vi "Lab Panel V5.28.vi"() -> ()   [LabVIEW 2013] (continued)
                  tunnel: w845 -> [_ w883]
                  tunnel: w844 -> [_ w882]
                  tunnel: w842 -> [w847 w881]
                  tunnel: w843 -> [_ w880]
                  tunnel: w841 -> [_ w879]
                  tunnel: [w846 w878] -> w840
                  tunnel: w838 -> [_ w877]
                  tunnel: w837 -> [_ w876]
                  tunnel: w836 -> [_ w875]
                  tunnel: w835 -> [_ w873]
                  frame False {
                    # "stop test"
                    n579 = stacked-sequence {
                      tunnel: w847 -> [w856 _]
                      tunnel: [w848 _] -> w846
                      frame #0 {
                        n580 = local read "DISP LAB01-2"() -> (w855:T4)
                        n581 = Unbundle(w855) -> ("CYCLE"=w853:dbl, "MINS"=w854:dbl)  [unwired: 1 out]
                        n582 = case shown="\"CHART TEST\", Default" w856 {
                          tunnel: w854 -> [_ _ w863]
                          tunnel: w853 -> [w861 w862 _]
                          tunnel: [w861 w862 w863] -> w852
                          frame "CHART TEST", Default {
                          }
                          frame "CYCLE TEST" {
                          }
                          frame "T-RISE TEST" {
                          }
                        }
                        n583 = local read "TDMS LAB01-2"() -> (w860:refnum<k34>)
                        n584 = Build Array("STOPPED") -> (w857:string[])
                        n585 = Build Array(w852) -> (w851:dbl[])
                        n586 = TDMS Write(0:w860, 5:"TEST RESULT", 7:w857, 9:w851) -> (4:w849:refnum<k34>, 15:w850:errorcluster)  [unwired: 2 in, 2 out]
                        n587 = TDMS Close(8:w850, 11:w849) -> (0:w848:errorcluster)  [unwired: 1 out]
                      }
                      frame #1 {
                        n588 = local read "DISP LAB01-2"() -> (w867:T4)
                        n589 = stacked-sequence {
                          tunnel: "LAB01-2" -> [w869 w871]
                          frame #0 {
                            n590 = call "sub vi - defrag tdms v1.vi"("panel id"=w869) -> ("error out"=w868:errorcluster)  [unwired: 10 in]
                            n591 = local write "data file error"(w868) -> ()
                          }
                          frame #1 {
                            n592 = call "Save data file (stop) v3.vi"("panel id"=w871) -> ("network file save error"=w870:errorcluster)  [unwired: 9 in, 1 out]
                            n593 = local write "RESULT LAB01-2"(FALSE) -> ()
                            n594 = local write "data file error"(w870) -> ()
                          }
                        }
                        n595 = Bundle(cluster=w867, "STATUS"="STOP") -> (w865:T4)  [unwired: 2 in]
                        n596 = local write "DISP LAB01-2"(w865) -> ()
                      }
                    }
                  }
                  frame True {
                    n597 = local read "SIG LAB01-2"() -> (w874:T2)
                    n598 = stacked-sequence {
                      seq-local: [w885 _] -> [_ w889]
                      tunnel: w883 -> [_ w899]
                      tunnel: w882 -> [_ w898]
                      tunnel: w881 -> [_ w897]
                      tunnel: w880 -> [_ w896]
                      tunnel: w879 -> [_ w895]
                      tunnel: [_ w894] -> w878
                      tunnel: w877 -> [_ w893]
                      tunnel: w876 -> [_ w892]
                      tunnel: w875 -> [_ w891]
                      tunnel: w874 -> [w884 w890]
                      tunnel: w873 -> [_ w888]
                      frame #0 {
                        n599 = Unbundle(w884) -> ("AMPS"=w887:dbl)  [unwired: 4 out]
                        n600 = call "Check For Amps on v1.vi"("ID"="LAB01-2", "amps"=w887) -> ("amps"=w885:bool)  [unwired: 9 in]
                      }
                      frame #1 {
                        n601 = case shown="True" w889 {
                          tunnel: w899 -> [_ w912]
                          tunnel: w898 -> [_ w911]
                          tunnel: w897 -> [_ w910]
                          tunnel: w896 -> [_ w909]
                          tunnel: w895 -> [_ w908]
                          tunnel: [errorcluster {"status"=FALSE, "code"=0, "source"=""} ("error out") w907] -> w894
                          tunnel: w893 -> [_ w906]
                          tunnel: w892 -> [_ w905]
                          tunnel: w891 -> [_ w904]
                          tunnel: w890 -> [_ w903]
                          tunnel: w888 -> [_ w902]
                          frame False {
                            w900 = FALSE
                            n602 = local write "RUN LAB01-2"(w900) -> ()
                            n603 = local write "run lab01-2"(w900) -> ()
                          }
                          frame True {
                            n604 = stacked-sequence {
                              seq-local: [w913 _ _ _ _] -> [_ w937 _ _ _]
                              tunnel: w912 -> [w918 _ _ _ _]
                              tunnel: w911 -> [w915 _ _ _ _]
                              tunnel: w910 -> [w928 _ _ _ _]
                              tunnel: w909 -> [w921 _ _ _ _]
                              tunnel: w908 -> [w916 _ _ _ _]
                              tunnel: [_ w932 _ _ _] -> w907
                              tunnel: w906 -> [_ _ _ w959 _]
                              tunnel: w905 -> [_ _ _ w958 _]
                              tunnel: w904 -> [_ _ _ w957 _]
                              tunnel: w903 -> [_ _ _ _ _]
                              tunnel: w902 -> [_ _ _ _ w972]
                              frame #0 {
                                w914 = "\\"
                                n605 = local read "SET LAB01-2"() -> (w923:T5)
                                n606 = case shown="\"CYCLE TEST\"" w928 {
                                tunnel: ["L01-2-CHART TEST-" "L01-2-CYCLE TEST-" "L01-2-T-RISE TEST-"] -> w924
                                frame "CHART TEST", Default {
                                }
                                frame "CYCLE TEST" {
                                }
                                frame "T-RISE TEST" {
                                }
                                }
                                n607 = Unbundle(w923) -> ("DESCRIPTION"=w922:string)  [unwired: 4 out]
                                n608 = Concatenate Strings(w918, "\\", w916, w914, w915, w914) -> (w925:string)
                                n609 = String To Path(string=w925) -> (path=w927:path)
                                n610 = Concatenate Strings(w925, w924, w922, "-", w921, ".tdms") -> (w913:string)
                                n611 = Create Folder(path (use dialog)=w927) -> (error out=w926:errorcluster)  [unwired: 2 in, 2 out]
                                n612 = call <vilib>:"Clear Errors.vi"("error in (no error)"=w926) -> ()  [unwired: 6 in, 1 out]
                                n613 = global write "Global 1.vi" "LAB01-2 FILE"(w913) -> ()
                              }
                              frame #1 {
                                (unwired) FALSE
                                n614 = String To Path(string=w937) -> (path=w933:path)
                                n615 = TDMS Open(6:FALSE, 10:T21."create or replace" ("operation (0:open)"), 11:w933) -> (0:w932:errorcluster, 3:→"TDMS LAB01-2":refnum<k34>)  [unwired: 4 in]
                              }
                              frame #2 {
                                n616 = local read "SET LAB01-2"() -> (w943:T5)
                                n617 = local read "TDMS LAB01-2"() -> (w954:refnum<k34>)
                                n618 = Build Array("Testers Name", "Description", "Set Test Cycles", "T-Rise minutes", "T-Rise Deg C") -> (w944:string[])
                                n619 = Unbundle(w943) -> ("NAME"=w942:string, "DESCRIPTION"=w941:string, "CYCLES"=w940:dbl, "T-RISE mins"=w939:dbl, "T-RISE deg C"=w938:dbl)
                                n620 = Number To Decimal String(number=w940) -> (decimal integer string=w953:string)  [unwired: 1 in]
                                n621 = Number To Decimal String(number=w939) -> (decimal integer string=w952:string)  [unwired: 1 in]
                                n622 = Number To Decimal String(number=w938) -> (decimal integer string=w951:string)  [unwired: 1 in]
                                n623 = Build Array(w942, w941, w953, w952, w951) -> (w950:string[])
                                n624 = TDMS Set Properties(5:w950, 7:w944, 11:w954) -> ()  [unwired: 3 in, 4 out]
                              }
                              frame #3 {
                                n625 = local read "DISP LAB01-2"() -> (w956:T4)
                                n626 = Concatenate Strings("LAB01-2  ", w959) -> (w960:string)
                                n627 = Two Button Dialog(message=w960, 1:w957, 2:w958) -> (T button?=w962:bool)
                                n628 = case shown="True" w962 {
                                tunnel: w956 -> [w969 w970]
                                tunnel: [w969 w970] -> w966
                                tunnel: [w968 w971] -> w965
                                tunnel: [w967 w971] -> w964
                                frame False {
                                n629 = Unbundle(w969) -> ("CYCLE"=w968:dbl, "MINS"=w967:dbl)  [unwired: 1 out]
                                }
                                frame True {
                                w971 = 0.0
                                }
                                }
                                n630 = Bundle(cluster=w966, "CYCLE"=w965, "MINS"=w964, "STATUS"="RUN") -> (w955:T4)
                                n631 = local write "DISP LAB01-2"(w955) -> ()
                              }
                              frame #4 {
                                n632 = local read "TEMP START LAB01-2"() -> (w974:cluster{"TL":dbl, "TN":dbl})
                                n633 = Bundle(cluster=w974, "TL"=w972, "TN"=w972) -> (w973:cluster{"TL":dbl, "TN":dbl})
                                n634 = local write "TEMP START LAB01-2"(w973) -> ()
                              }
                            }
                          }
                        }
                      }
                    }
                  }
                }
              }
              event "RUN LAB02-1": Value Change {
                n635 = event-data() -> ("NewVal"=w980:bool)  [unwired: 1 in, 5 out]
                n636 = local read "SIG LAB02-1"() -> (w976:T2)
                n637 = case shown="True" w980 {
                  tunnel: w986 -> [_ w1024]
                  tunnel: w985 -> [_ w1023]
                  tunnel: w983 -> [w988 w1022]
                  tunnel: w984 -> [_ w1021]
                  tunnel: w982 -> [_ w1020]
                  tunnel: [w987 w1019] -> w981
                  tunnel: w979 -> [_ w1018]
                  tunnel: w978 -> [_ w1017]
                  tunnel: w977 -> [_ w1016]
                  tunnel: w976 -> [_ w1015]
                  tunnel: w975 -> [_ w1014]
                  frame False {
                    # "stop test"
                    n638 = stacked-sequence {
                      tunnel: w988 -> [w997 _]
                      tunnel: [w989 _] -> w987
                      frame #0 {
                        n639 = local read "DISP LAB02-1"() -> (w996:T4)
                        n640 = Unbundle(w996) -> ("CYCLE"=w994:dbl, "MINS"=w995:dbl)  [unwired: 1 out]
                        n641 = case shown="\"CYCLE TEST\"" w997 {
                          tunnel: w995 -> [_ _ w1004]
                          tunnel: w994 -> [w1002 w1003 _]
                          tunnel: [w1002 w1003 w1004] -> w993
                          frame "CHART TEST", Default {
                          }
                          frame "CYCLE TEST" {
                          }
                          frame "T-RISE TEST" {
                          }
                        }
                        n642 = local read "TDMS LAB02-1"() -> (w1001:refnum<k34>)
                        n643 = Build Array("STOPPED") -> (w998:string[])
                        n644 = Build Array(w993) -> (w992:dbl[])
                        n645 = TDMS Write(0:w1001, 5:"TEST RESULT", 7:w998, 9:w992) -> (4:w990:refnum<k34>, 15:w991:errorcluster)  [unwired: 2 in, 2 out]
                        n646 = TDMS Close(8:w991, 11:w990) -> (0:w989:errorcluster)  [unwired: 1 out]
                      }
                      frame #1 {
                        n647 = local read "DISP LAB02-1"() -> (w1008:T4)
                        n648 = stacked-sequence {
                          tunnel: "LAB02-1" -> [w1010 w1012]
                          frame #0 {
                            n649 = call "sub vi - defrag tdms v1.vi"("panel id"=w1010) -> ("error out"=w1009:errorcluster)  [unwired: 10 in]
                            n650 = local write "data file error"(w1009) -> ()
                          }
                          frame #1 {
                            n651 = local write "RESULT LAB02-1"(FALSE) -> ()
                            n652 = call "Save data file (stop) v3.vi"("panel id"=w1012) -> ("network file save error"=w1011:errorcluster)  [unwired: 9 in, 1 out]
                            n653 = local write "data file error"(w1011) -> ()
                          }
                        }
                        n654 = Bundle(cluster=w1008, "STATUS"="STOP") -> (w1006:T4)  [unwired: 2 in]
                        n655 = local write "DISP LAB02-1"(w1006) -> ()
                      }
                    }
                  }
                  frame True {
                    n656 = stacked-sequence {
                      seq-local: [w1026 _] -> [_ w1030]
                      tunnel: w1024 -> [_ w1040]
                      tunnel: w1023 -> [_ w1039]
                      tunnel: w1022 -> [_ w1038]
                      tunnel: w1021 -> [_ w1037]
                      tunnel: w1020 -> [_ w1036]
                      tunnel: [_ w1035] -> w1019
                      tunnel: w1018 -> [_ w1034]
                      tunnel: w1017 -> [_ w1033]
                      tunnel: w1016 -> [_ w1032]
                      tunnel: w1015 -> [w1025 w1031]
                      tunnel: w1014 -> [_ w1029]
                      frame #0 {
                        n657 = Unbundle(w1025) -> ("AMPS"=w1028:dbl)  [unwired: 4 out]
                        n658 = call "Check For Amps on v1.vi"("ID"="LAB02-1", "amps"=w1028) -> ("amps"=w1026:bool)  [unwired: 9 in]
                      }
                      frame #1 {
                        n659 = case shown="True" w1030 {
                          tunnel: w1040 -> [_ w1053]
                          tunnel: w1039 -> [_ w1052]
                          tunnel: w1038 -> [_ w1051]
                          tunnel: w1037 -> [_ w1050]
                          tunnel: w1036 -> [_ w1049]
                          tunnel: [errorcluster {"status"=FALSE, "code"=0, "source"=""} ("error out") w1048] -> w1035
                          tunnel: w1034 -> [_ w1047]
                          tunnel: w1033 -> [_ w1046]
                          tunnel: w1032 -> [_ w1045]
                          tunnel: w1031 -> [_ w1044]
                          tunnel: w1029 -> [_ w1043]
                          frame False {
                            w1042 = FALSE
                            n660 = local write "RUN LAB02-1"(w1042) -> ()
                            n661 = local write "run lab02-1"(w1042) -> ()
                          }
                          frame True {
                            n662 = stacked-sequence {
                              seq-local: [w1054 _ _ _ _] -> [_ w1078 _ _ _]
                              tunnel: w1053 -> [w1059 _ _ _ _]
                              tunnel: w1052 -> [w1056 _ _ _ _]
                              tunnel: w1051 -> [w1069 _ _ _ _]
                              tunnel: w1050 -> [w1062 _ _ _ _]
                              tunnel: w1049 -> [w1057 _ _ _ _]
                              tunnel: [_ w1073 _ _ _] -> w1048
                              tunnel: w1047 -> [_ _ _ w1099 _]
                              tunnel: w1046 -> [_ _ _ w1098 _]
                              tunnel: w1045 -> [_ _ _ w1097 _]
                              tunnel: w1044 -> [_ _ _ _ _]
                              tunnel: w1043 -> [_ _ _ _ w1113]
                              frame #0 {
                                w1055 = "\\"
                                n663 = local read "SET LAB02-1"() -> (w1064:T5)
                                n664 = case shown="\"CYCLE TEST\"" w1069 {
                                tunnel: ["L02-1-CHART TEST-" "L02-1-CYCLE TEST-" "L02-1-T-RISE TEST-"] -> w1065
                                frame "CHART TEST", Default {
                                }
                                frame "CYCLE TEST" {
                                }
                                frame "T-RISE TEST" {
                                }
                                }
                                n665 = Unbundle(w1064) -> ("DESCRIPTION"=w1063:string)  [unwired: 4 out]
                                n666 = Concatenate Strings(w1059, "\\", w1057, w1055, w1056, w1055) -> (w1066:string)
                                n667 = String To Path(string=w1066) -> (path=w1068:path)
                                n668 = Concatenate Strings(w1066, w1065, w1063, "-", w1062, ".tdms") -> (w1054:string)
                                n669 = Create Folder(path (use dialog)=w1068) -> (error out=w1067:errorcluster)  [unwired: 2 in, 2 out]
                                n670 = global write "Global 1.vi" "LAB02-1 FILE"(w1054) -> ()
                                n671 = call <vilib>:"Clear Errors.vi"("error in (no error)"=w1067) -> ()  [unwired: 6 in, 1 out]
                              }
                              frame #1 {
                                (unwired) FALSE
                                n672 = String To Path(string=w1078) -> (path=w1074:path)
                                n673 = TDMS Open(6:FALSE, 10:T21."create or replace" ("operation (0:open)"), 11:w1074) -> (0:w1073:errorcluster, 3:→"TDMS LAB02-1":refnum<k34>)  [unwired: 4 in]
                              }
                              frame #2 {
                                n674 = local read "SET LAB02-1"() -> (w1084:T5)
                                n675 = local read "TDMS LAB02-1"() -> (w1095:refnum<k34>)
                                n676 = Build Array("Testers Name", "Description", "Set Test Cycles", "T-Rise minutes", "T-Rise Deg C") -> (w1085:string[])
                                n677 = Unbundle(w1084) -> ("NAME"=w1083:string, "DESCRIPTION"=w1082:string, "CYCLES"=w1081:dbl, "T-RISE mins"=w1080:dbl, "T-RISE deg C"=w1079:dbl)
                                n678 = Number To Decimal String(number=w1081) -> (decimal integer string=w1094:string)  [unwired: 1 in]
                                n679 = Number To Decimal String(number=w1080) -> (decimal integer string=w1093:string)  [unwired: 1 in]
                                n680 = Number To Decimal String(number=w1079) -> (decimal integer string=w1092:string)  [unwired: 1 in]
                                n681 = Build Array(w1083, w1082, w1094, w1093, w1092) -> (w1091:string[])
                                n682 = TDMS Set Properties(5:w1091, 7:w1085, 11:w1095) -> ()  [unwired: 3 in, 4 out]
                              }
                              frame #3 {
                                n683 = local read "DISP LAB02-1"() -> (w1100:T4)
                                n684 = Concatenate Strings("LAB02-1  ", w1099) -> (w1101:string)
                                n685 = Two Button Dialog(message=w1101, 1:w1097, 2:w1098) -> (T button?=w1103:bool)
                                n686 = case shown="True" w1103 {
                                tunnel: w1100 -> [w1110 w1111]
                                tunnel: [w1110 w1111] -> w1107
                                tunnel: [w1109 w1112] -> w1106
                                tunnel: [w1108 w1112] -> w1105
                                frame False {
                                n687 = Unbundle(w1110) -> ("CYCLE"=w1109:dbl, "MINS"=w1108:dbl)  [unwired: 1 out]
                                }
                                frame True {
                                w1112 = 0.0
                                }
                                }
                                n688 = Bundle(cluster=w1107, "CYCLE"=w1106, "MINS"=w1105, "STATUS"="RUN") -> (w1096:T4)
                                n689 = local write "DISP LAB02-1"(w1096) -> ()
                              }
                              frame #4 {
                                n690 = local read "TEMP START LAB02-1"() -> (w1115:cluster{"TL":dbl, "TN":dbl})
                                n691 = Bundle(cluster=w1115, "TL"=w1113, "TN"=w1113) -> (w1114:cluster{"TL":dbl, "TN":dbl})
                                n692 = local write "TEMP START LAB02-1"(w1114) -> ()
                              }
                            }
                          }
                        }
                      }
                    }
                  }
                }
                n693 = local write "run lab02-1"(w980) -> ()
              }
              event "RUN LAB02-2": Value Change {
                n694 = event-data() -> ("NewVal"=w1120:bool)  [unwired: 1 in, 5 out]
                n695 = local write "run lab02-2"(w1120) -> ()
                n696 = case shown="True" w1120 {
                  tunnel: w1126 -> [_ w1164]
                  tunnel: w1125 -> [_ w1163]
                  tunnel: w1123 -> [w1128 w1162]
                  tunnel: w1124 -> [_ w1161]
                  tunnel: w1122 -> [_ w1160]
                  tunnel: [w1127 w1159] -> w1121
                  tunnel: w1119 -> [_ w1158]
                  tunnel: w1118 -> [_ w1157]
                  tunnel: w1117 -> [_ w1156]
                  tunnel: w1116 -> [_ w1154]
                  frame False {
                    # "stop test"
                    n697 = stacked-sequence {
                      tunnel: w1128 -> [w1137 _]
                      tunnel: [w1129 _] -> w1127
                      frame #0 {
                        n698 = local read "DISP LAB02-2"() -> (w1136:T4)
                        n699 = Unbundle(w1136) -> ("CYCLE"=w1134:dbl, "MINS"=w1135:dbl)  [unwired: 1 out]
                        n700 = case shown="\"CYCLE TEST\"" w1137 {
                          tunnel: w1135 -> [_ _ w1144]
                          tunnel: w1134 -> [w1142 w1143 _]
                          tunnel: [w1142 w1143 w1144] -> w1133
                          frame "CHART TEST", Default {
                          }
                          frame "CYCLE TEST" {
                          }
                          frame "T-RISE TEST" {
                          }
                        }
                        n701 = local read "TDMS LAB02-2"() -> (w1141:refnum<k34>)
                        n702 = Build Array("STOPPED") -> (w1138:string[])
                        n703 = Build Array(w1133) -> (w1132:dbl[])
                        n704 = TDMS Write(0:w1141, 5:"TEST RESULT", 7:w1138, 9:w1132) -> (4:w1130:refnum<k34>, 15:w1131:errorcluster)  [unwired: 2 in, 2 out]
                        n705 = TDMS Close(8:w1131, 11:w1130) -> (0:w1129:errorcluster)  [unwired: 1 out]
                      }
                      frame #1 {
                        n706 = local read "DISP LAB02-2"() -> (w1148:T4)
                        n707 = stacked-sequence {
                          tunnel: "LAB02-2" -> [w1150 w1152]
                          frame #0 {
                            n708 = call "sub vi - defrag tdms v1.vi"("panel id"=w1150) -> ("error out"=w1149:errorcluster)  [unwired: 10 in]
                            n709 = local write "data file error"(w1149) -> ()
                          }
                          frame #1 {
                            n710 = call "Save data file (stop) v3.vi"("panel id"=w1152) -> ("network file save error"=w1151:errorcluster)  [unwired: 9 in, 1 out]
                            n711 = local write "RESULT LAB02-2"(FALSE) -> ()
                            n712 = local write "data file error"(w1151) -> ()
                          }
                        }
                        n713 = Bundle(cluster=w1148, "STATUS"="STOP") -> (w1146:T4)  [unwired: 2 in]
                        n714 = local write "DISP LAB02-2"(w1146) -> ()
                      }
                    }
                  }
                  frame True {
                    n715 = local read "SIG LAB02-2"() -> (w1155:T2)
                    n716 = stacked-sequence {
                      seq-local: [w1166 _] -> [_ w1170]
                      tunnel: w1164 -> [_ w1180]
                      tunnel: w1163 -> [_ w1179]
                      tunnel: w1162 -> [_ w1178]
                      tunnel: w1161 -> [_ w1177]
                      tunnel: w1160 -> [_ w1176]
                      tunnel: [_ w1175] -> w1159
                      tunnel: w1158 -> [_ w1174]
                      tunnel: w1157 -> [_ w1173]
                      tunnel: w1156 -> [_ w1172]
                      tunnel: w1155 -> [w1165 w1171]
                      tunnel: w1154 -> [_ w1169]
                      frame #0 {
                        n717 = Unbundle(w1165) -> ("AMPS"=w1168:dbl)  [unwired: 4 out]
                        n718 = call "Check For Amps on v1.vi"("ID"="LAB02-2", "amps"=w1168) -> ("amps"=w1166:bool)  [unwired: 9 in]
                      }
                      frame #1 {
                        n719 = case shown="True" w1170 {
                          tunnel: w1180 -> [_ w1193]
                          tunnel: w1179 -> [_ w1192]
                          tunnel: w1178 -> [_ w1191]
                          tunnel: w1177 -> [_ w1190]
                          tunnel: w1176 -> [_ w1189]
                          tunnel: [errorcluster {"status"=FALSE, "code"=0, "source"=""} ("error out") w1188] -> w1175
                          tunnel: w1174 -> [_ w1187]
                          tunnel: w1173 -> [_ w1186]
                          tunnel: w1172 -> [_ w1185]
                          tunnel: w1171 -> [_ w1184]
                          tunnel: w1169 -> [_ w1183]
                          frame False {
                            w1181 = FALSE
                            n720 = local write "RUN LAB02-2"(w1181) -> ()
                            n721 = local write "run lab02-2"(w1181) -> ()
                          }
                          frame True {
                            n722 = stacked-sequence {
                              seq-local: [w1194 _ _ _ _] -> [_ w1218 _ _ _]
                              tunnel: w1193 -> [w1199 _ _ _ _]
                              tunnel: w1192 -> [w1196 _ _ _ _]
                              tunnel: w1191 -> [w1209 _ _ _ _]
                              tunnel: w1190 -> [w1202 _ _ _ _]
                              tunnel: w1189 -> [w1197 _ _ _ _]
                              tunnel: [_ w1213 _ _ _] -> w1188
                              tunnel: w1187 -> [_ _ _ w1239 _]
                              tunnel: w1186 -> [_ _ _ w1238 _]
                              tunnel: w1185 -> [_ _ _ w1237 _]
                              tunnel: w1184 -> [_ _ _ _ _]
                              tunnel: w1183 -> [_ _ _ _ w1253]
                              frame #0 {
                                w1195 = "\\"
                                n723 = local read "SET LAB02-2"() -> (w1204:T5)
                                n724 = case shown="\"CYCLE TEST\"" w1209 {
                                tunnel: ["L02-2-CHART TEST-" "L02-2-CYCLE TEST-" "L02-2-T-RISE TEST-"] -> w1205
                                frame "CHART TEST", Default {
                                }
                                frame "CYCLE TEST" {
                                }
                                frame "T-RISE TEST" {
                                }
                                }
                                n725 = Unbundle(w1204) -> ("DESCRIPTION"=w1203:string)  [unwired: 4 out]
                                n726 = Concatenate Strings(w1199, "\\", w1197, w1195, w1196, w1195) -> (w1206:string)
                                n727 = String To Path(string=w1206) -> (path=w1208:path)
                                n728 = Concatenate Strings(w1206, w1205, w1203, "-", w1202, ".tdms") -> (w1194:string)
                                n729 = Create Folder(path (use dialog)=w1208) -> (error out=w1207:errorcluster)  [unwired: 2 in, 2 out]
                                n730 = global write "Global 1.vi" "LAB02-2 FILE"(w1194) -> ()
                                n731 = call <vilib>:"Clear Errors.vi"("error in (no error)"=w1207) -> ()  [unwired: 6 in, 1 out]
                              }
                              frame #1 {
                                (unwired) FALSE
                                n732 = String To Path(string=w1218) -> (path=w1214:path)
                                n733 = TDMS Open(6:FALSE, 10:T21."create or replace" ("operation (0:open)"), 11:w1214) -> (0:w1213:errorcluster, 3:→"TDMS LAB02-2":refnum<k34>)  [unwired: 4 in]
                              }
                              frame #2 {
                                n734 = local read "SET LAB02-2"() -> (w1224:T5)
                                n735 = local read "TDMS LAB02-2"() -> (w1235:refnum<k34>)
                                n736 = Build Array("Testers Name", "Description", "Set Test Cycles", "T-Rise minutes", "T-Rise Deg C") -> (w1225:string[])
                                n737 = Unbundle(w1224) -> ("NAME"=w1223:string, "DESCRIPTION"=w1222:string, "CYCLES"=w1221:dbl, "T-RISE mins"=w1220:dbl, "T-RISE deg C"=w1219:dbl)
                                n738 = Number To Decimal String(number=w1221) -> (decimal integer string=w1234:string)  [unwired: 1 in]
                                n739 = Number To Decimal String(number=w1220) -> (decimal integer string=w1233:string)  [unwired: 1 in]
                                n740 = Number To Decimal String(number=w1219) -> (decimal integer string=w1232:string)  [unwired: 1 in]
                                n741 = Build Array(w1223, w1222, w1234, w1233, w1232) -> (w1231:string[])
                                n742 = TDMS Set Properties(5:w1231, 7:w1225, 11:w1235) -> ()  [unwired: 3 in, 4 out]
                              }
                              frame #3 {
                                n743 = local read "DISP LAB02-2"() -> (w1240:T4)
                                n744 = Concatenate Strings("LAB02-2  ", w1239) -> (w1241:string)
                                n745 = Two Button Dialog(message=w1241, 1:w1237, 2:w1238) -> (T button?=w1243:bool)
                                n746 = case shown="True" w1243 {
                                tunnel: w1240 -> [w1250 w1251]
                                tunnel: [w1250 w1251] -> w1247
                                tunnel: [w1249 w1252] -> w1246
                                tunnel: [w1248 w1252] -> w1245
                                frame False {
                                n747 = Unbundle(w1250) -> ("CYCLE"=w1249:dbl, "MINS"=w1248:dbl)  [unwired: 1 out]
                                }
                                frame True {
                                w1252 = 0.0
                                }
                                }
                                n748 = Bundle(cluster=w1247, "CYCLE"=w1246, "MINS"=w1245, "STATUS"="RUN") -> (w1236:T4)
                                n749 = local write "DISP LAB02-2"(w1236) -> ()
                              }
                              frame #4 {
                                n750 = local read "TEMP START LAB02-2"() -> (w1255:cluster{"TL":dbl, "TN":dbl})
                                n751 = Bundle(cluster=w1255, "TL"=w1253, "TN"=w1253) -> (w1254:cluster{"TL":dbl, "TN":dbl})
                                n752 = local write "TEMP START LAB02-2"(w1254) -> ()
                              }
                            }
                          }
                        }
                      }
                    }
                  }
                }
              }
              event "RUN LAB03-1": Value Change {
                n753 = event-data() -> ("NewVal"=w1260:bool)  [unwired: 1 in, 5 out]
                n754 = local write "run lab03-1"(w1260) -> ()
                n755 = case shown="True" w1260 {
                  tunnel: w1266 -> [_ w1304]
                  tunnel: w1265 -> [_ w1303]
                  tunnel: w1263 -> [w1268 w1302]
                  tunnel: w1264 -> [_ w1301]
                  tunnel: w1262 -> [_ w1300]
                  tunnel: [w1267 w1299] -> w1261
                  tunnel: w1259 -> [_ w1298]
                  tunnel: w1258 -> [_ w1297]
                  tunnel: w1257 -> [_ w1296]
                  tunnel: w1256 -> [_ w1294]
                  frame False {
                    # "stop test"
                    n756 = stacked-sequence {
                      tunnel: w1268 -> [w1277 _]
                      tunnel: [w1269 _] -> w1267
                      frame #0 {
                        n757 = local read "DISP LAB03-1"() -> (w1276:T4)
                        n758 = Unbundle(w1276) -> ("CYCLE"=w1274:dbl, "MINS"=w1275:dbl)  [unwired: 1 out]
                        n759 = case shown="\"CYCLE TEST\"" w1277 {
                          tunnel: w1275 -> [_ _ w1284]
                          tunnel: w1274 -> [w1282 w1283 _]
                          tunnel: [w1282 w1283 w1284] -> w1273
                          frame "CHART TEST", Default {
                          }
                          frame "CYCLE TEST" {
                          }
                          frame "T-RISE TEST" {
                          }
                        }
                        n760 = local read "TDMS LAB03-1"() -> (w1281:refnum<k34>)
                        n761 = Build Array("STOPPED") -> (w1278:string[])
                        n762 = Build Array(w1273) -> (w1272:dbl[])
                        n763 = TDMS Write(0:w1281, 5:"TEST RESULT", 7:w1278, 9:w1272) -> (4:w1270:refnum<k34>, 15:w1271:errorcluster)  [unwired: 2 in, 2 out]
                        n764 = TDMS Close(8:w1271, 11:w1270) -> (0:w1269:errorcluster)  [unwired: 1 out]
                      }
                      frame #1 {
                        n765 = local read "DISP LAB03-1"() -> (w1288:T4)
                        n766 = stacked-sequence {
                          tunnel: "LAB03-1" -> [w1290 w1292]
                          frame #0 {
                            n767 = call "sub vi - defrag tdms v1.vi"("panel id"=w1290) -> ("error out"=w1289:errorcluster)  [unwired: 10 in]
                            n768 = local write "data file error"(w1289) -> ()
                          }
                          frame #1 {
                            n769 = call "Save data file (stop) v3.vi"("panel id"=w1292) -> ("network file save error"=w1291:errorcluster)  [unwired: 9 in, 1 out]
                            n770 = local write "RESULT LAB03-1"(FALSE) -> ()
                            n771 = local write "data file error"(w1291) -> ()
                          }
                        }
                        n772 = Bundle(cluster=w1288, "STATUS"="STOP") -> (w1286:T4)  [unwired: 2 in]
                        n773 = local write "DISP LAB03-1"(w1286) -> ()
                      }
                    }
                  }
                  frame True {
                    n774 = local read "SIG LAB03-1"() -> (w1295:T2)
                    n775 = stacked-sequence {
                      seq-local: [w1306 _] -> [_ w1310]
                      tunnel: w1304 -> [_ w1320]
                      tunnel: w1303 -> [_ w1319]
                      tunnel: w1302 -> [_ w1318]
                      tunnel: w1301 -> [_ w1317]
                      tunnel: w1300 -> [_ w1316]
                      tunnel: [_ w1315] -> w1299
                      tunnel: w1298 -> [_ w1314]
                      tunnel: w1297 -> [_ w1313]
                      tunnel: w1296 -> [_ w1312]
                      tunnel: w1295 -> [w1305 w1311]
                      tunnel: w1294 -> [_ w1309]
                      frame #0 {
                        n776 = Unbundle(w1305) -> ("AMPS"=w1308:dbl)  [unwired: 4 out]
                        n777 = call "Check For Amps on v1.vi"("ID"="LAB03-1", "amps"=w1308) -> ("amps"=w1306:bool)  [unwired: 9 in]
                      }
                      frame #1 {
                        n778 = case shown="True" w1310 {
                          tunnel: w1320 -> [_ w1333]
                          tunnel: w1319 -> [_ w1332]
                          tunnel: w1318 -> [_ w1331]
                          tunnel: w1317 -> [_ w1330]
                          tunnel: w1316 -> [_ w1329]
                          tunnel: [errorcluster {"status"=FALSE, "code"=0, "source"=""} ("error out") w1328] -> w1315
                          tunnel: w1314 -> [_ w1327]
                          tunnel: w1313 -> [_ w1326]
                          tunnel: w1312 -> [_ w1325]
                          tunnel: w1311 -> [_ w1324]
                          tunnel: w1309 -> [_ w1323]
                          frame False {
                            w1321 = FALSE
                            n779 = local write "RUN LAB03-1"(w1321) -> ()
                            n780 = local write "run lab03-1"(w1321) -> ()
                          }
                          frame True {
                            n781 = stacked-sequence {
                              seq-local: [w1334 _ _ _ _] -> [_ w1358 _ _ _]
                              tunnel: w1333 -> [w1339 _ _ _ _]
                              tunnel: w1332 -> [w1336 _ _ _ _]
                              tunnel: w1331 -> [w1349 _ _ _ _]
                              tunnel: w1330 -> [w1342 _ _ _ _]
                              tunnel: w1329 -> [w1337 _ _ _ _]
                              tunnel: [_ w1353 _ _ _] -> w1328
                              tunnel: w1327 -> [_ _ _ w1378 _]
                              tunnel: w1326 -> [_ _ _ w1377 _]
                              tunnel: w1325 -> [_ _ _ w1376 _]
                              tunnel: w1324 -> [_ _ _ _ _]
                              tunnel: w1323 -> [_ _ _ _ w1393]
                              frame #0 {
                                w1335 = "\\"
                                n782 = local read "SET LAB03-1"() -> (w1344:T5)
                                n783 = case shown="\"T-RISE TEST\"" w1349 {
                                tunnel: ["L03-1-CHART TEST-" "L03-1-CYCLE TEST-" "L03-1-T-RISE TEST-"] -> w1345
                                frame "CHART TEST", Default {
                                }
                                frame "CYCLE TEST" {
                                }
                                frame "T-RISE TEST" {
                                }
                                }
                                n784 = Unbundle(w1344) -> ("DESCRIPTION"=w1343:string)  [unwired: 4 out]
                                n785 = Concatenate Strings(w1339, "\\", w1337, w1335, w1336, w1335) -> (w1346:string)
                                n786 = String To Path(string=w1346) -> (path=w1348:path)
                                n787 = Concatenate Strings(w1346, w1345, w1343, "-", w1342, ".tdms") -> (w1334:string)
                                n788 = Create Folder(path (use dialog)=w1348) -> (error out=w1347:errorcluster)  [unwired: 2 in, 2 out]
                                n789 = global write "Global 1.vi" "LAB03-1 FILE"(w1334) -> ()
                                n790 = call <vilib>:"Clear Errors.vi"("error in (no error)"=w1347) -> ()  [unwired: 6 in, 1 out]
                              }
                              frame #1 {
                                (unwired) FALSE
                                n791 = String To Path(string=w1358) -> (path=w1354:path)
                                n792 = TDMS Open(6:FALSE, 10:T21."create or replace" ("operation (0:open)"), 11:w1354) -> (0:w1353:errorcluster, 3:→"TDMS LAB03-1":refnum<k34>)  [unwired: 4 in]
                              }
                              frame #2 {
                                n793 = local read "SET LAB03-1"() -> (w1364:T5)
                                n794 = local read "TDMS LAB03-1"() -> (w1375:refnum<k34>)
                                n795 = Build Array("Testers Name", "Description", "Set Test Cycles", "T-Rise minutes", "T-Rise Deg C") -> (w1365:string[])
                                n796 = Unbundle(w1364) -> ("NAME"=w1363:string, "DESCRIPTION"=w1362:string, "CYCLES"=w1361:dbl, "T-RISE mins"=w1360:dbl, "T-RISE deg C"=w1359:dbl)
                                n797 = Number To Decimal String(number=w1361) -> (decimal integer string=w1374:string)  [unwired: 1 in]
                                n798 = Number To Decimal String(number=w1360) -> (decimal integer string=w1373:string)  [unwired: 1 in]
                                n799 = Number To Decimal String(number=w1359) -> (decimal integer string=w1372:string)  [unwired: 1 in]
                                n800 = Build Array(w1363, w1362, w1374, w1373, w1372) -> (w1371:string[])
                                n801 = TDMS Set Properties(5:w1371, 7:w1365, 11:w1375) -> ()  [unwired: 3 in, 4 out]
                              }
                              frame #3 {
                                n802 = local read "DISP LAB03-1"() -> (w1380:T4)
                                n803 = Concatenate Strings("LAB03-1  ", w1378) -> (w1381:string)
                                n804 = Two Button Dialog(message=w1381, 1:w1376, 2:w1377) -> (T button?=w1383:bool)
                                n805 = case shown="True" w1383 {
                                tunnel: w1380 -> [w1390 w1391]
                                tunnel: [w1390 w1391] -> w1387
                                tunnel: [w1389 w1392] -> w1386
                                tunnel: [w1388 w1392] -> w1385
                                frame False {
                                n806 = Unbundle(w1390) -> ("CYCLE"=w1389:dbl, "MINS"=w1388:dbl)  [unwired: 1 out]
                                }
                                frame True {
                                w1392 = 0.0
                                }
                                }
                                n807 = Bundle(cluster=w1387, "CYCLE"=w1386, "MINS"=w1385, "STATUS"="RUN") -> (w1379:T4)
                                n808 = local write "DISP LAB03-1"(w1379) -> ()
                              }
                              frame #4 {
                                n809 = local read "TEMP START LAB03-1"() -> (w1395:cluster{"TL":dbl, "TN":dbl})
                                n810 = Bundle(cluster=w1395, "TL"=w1393, "TN"=w1393) -> (w1394:cluster{"TL":dbl, "TN":dbl})
                                n811 = local write "TEMP START LAB03-1"(w1394) -> ()
                              }
                            }
                          }
                        }
                      }
                    }
                  }
                }
              }
              event "RUN LAB03-2": Value Change {
                n812 = event-data() -> ("NewVal"=w1400:bool)  [unwired: 1 in, 5 out]
                n813 = local write "run lab03-2"(w1400) -> ()
                n814 = case shown="True" w1400 {
                  tunnel: w1406 -> [_ w1444]
                  tunnel: w1405 -> [_ w1443]
                  tunnel: w1403 -> [w1408 w1442]
                  tunnel: w1404 -> [_ w1441]
                  tunnel: w1402 -> [_ w1440]
                  tunnel: [w1407 w1439] -> w1401
                  tunnel: w1399 -> [_ w1438]
                  tunnel: w1398 -> [_ w1437]
                  tunnel: w1397 -> [_ w1436]
                  tunnel: w1396 -> [_ w1434]
                  frame False {
                    # "stop test"
                    n815 = stacked-sequence {
                      tunnel: w1408 -> [w1417 _]
                      tunnel: [w1409 _] -> w1407
                      frame #0 {
                        n816 = local read "DISP LAB03-2"() -> (w1416:T4)
                        n817 = Unbundle(w1416) -> ("CYCLE"=w1414:dbl, "MINS"=w1415:dbl)  [unwired: 1 out]
                        n818 = case shown="\"CYCLE TEST\"" w1417 {
                          tunnel: w1415 -> [_ _ w1424]
                          tunnel: w1414 -> [w1422 w1423 _]
                          tunnel: [w1422 w1423 w1424] -> w1413
                          frame "CHART TEST", Default {
                          }
                          frame "CYCLE TEST" {
                          }
                          frame "T-RISE TEST" {
                          }
                        }
                        n819 = local read "TDMS LAB03-2"() -> (w1421:refnum<k34>)
                        n820 = Build Array("STOPPED") -> (w1418:string[])
                        n821 = Build Array(w1413) -> (w1412:dbl[])
                        n822 = TDMS Write(0:w1421, 5:"TEST RESULT", 7:w1418, 9:w1412) -> (4:w1410:refnum<k34>, 15:w1411:errorcluster)  [unwired: 2 in, 2 out]
                        n823 = TDMS Close(8:w1411, 11:w1410) -> (0:w1409:errorcluster)  [unwired: 1 out]
                      }
                      frame #1 {
                        n824 = local read "DISP LAB03-2"() -> (w1428:T4)
                        n825 = stacked-sequence {
                          tunnel: "LAB03-2" -> [w1430 w1432]
                          frame #0 {
                            n826 = call "sub vi - defrag tdms v1.vi"("panel id"=w1430) -> ("error out"=w1429:errorcluster)  [unwired: 10 in]
                            n827 = local write "data file error"(w1429) -> ()
                          }
                          frame #1 {
                            n828 = call "Save data file (stop) v3.vi"("panel id"=w1432) -> ("network file save error"=w1431:errorcluster)  [unwired: 9 in, 1 out]
                            n829 = local write "RESULT LAB03-2"(FALSE) -> ()
                            n830 = local write "data file error"(w1431) -> ()
                          }
                        }
                        n831 = Bundle(cluster=w1428, "STATUS"="STOP") -> (w1426:T4)  [unwired: 2 in]
                        n832 = local write "DISP LAB03-2"(w1426) -> ()
                      }
                    }
                  }
                  frame True {
                    n833 = local read "SIG LAB03-2"() -> (w1435:T2)
                    n834 = stacked-sequence {
                      seq-local: [w1446 _] -> [_ w1450]
                      tunnel: w1444 -> [_ w1460]
                      tunnel: w1443 -> [_ w1459]
                      tunnel: w1442 -> [_ w1458]
                      tunnel: w1441 -> [_ w1457]
                      tunnel: w1440 -> [_ w1456]
                      tunnel: [_ w1455] -> w1439
                      tunnel: w1438 -> [_ w1454]
                      tunnel: w1437 -> [_ w1453]
                      tunnel: w1436 -> [_ w1452]
                      tunnel: w1435 -> [w1445 w1451]
                      tunnel: w1434 -> [_ w1449]
                      frame #0 {
                        n835 = Unbundle(w1445) -> ("AMPS"=w1448:dbl)  [unwired: 4 out]
                        n836 = call "Check For Amps on v1.vi"("ID"="LAB03-2", "amps"=w1448) -> ("amps"=w1446:bool)  [unwired: 9 in]
                      }
                      frame #1 {
                        n837 = case shown="True" w1450 {
                          tunnel: w1460 -> [_ w1473]
                          tunnel: w1459 -> [_ w1472]
                          tunnel: w1458 -> [_ w1471]
                          tunnel: w1457 -> [_ w1470]
                          tunnel: w1456 -> [_ w1469]
                          tunnel: [errorcluster {"status"=FALSE, "code"=0, "source"=""} ("error out") w1468] -> w1455
                          tunnel: w1454 -> [_ w1467]
                          tunnel: w1453 -> [_ w1466]
                          tunnel: w1452 -> [_ w1465]
                          tunnel: w1451 -> [_ w1464]
                          tunnel: w1449 -> [_ w1463]
                          frame False {
                            w1461 = FALSE
                            n838 = local write "RUN LAB03-2"(w1461) -> ()
                            n839 = local write "run lab03-2"(w1461) -> ()
                          }
                          frame True {
                            n840 = stacked-sequence {
                              seq-local: [w1474 _ _ _ _] -> [_ w1498 _ _ _]
                              tunnel: w1473 -> [w1479 _ _ _ _]
                              tunnel: w1472 -> [w1476 _ _ _ _]
                              tunnel: w1471 -> [w1489 _ _ _ _]
                              tunnel: w1470 -> [w1482 _ _ _ _]
                              tunnel: w1469 -> [w1477 _ _ _ _]
                              tunnel: [_ w1493 _ _ _] -> w1468
                              tunnel: w1467 -> [_ _ _ w1519 _]
                              tunnel: w1466 -> [_ _ _ w1518 _]
                              tunnel: w1465 -> [_ _ _ w1517 _]
                              tunnel: w1464 -> [_ _ _ _ _]
                              tunnel: w1463 -> [_ _ _ _ w1533]
                              frame #0 {
                                w1475 = "\\"
                                n841 = local read "SET LAB03-2"() -> (w1484:T5)
                                n842 = case shown="\"T-RISE TEST\"" w1489 {
                                tunnel: ["L03-2-CHART TEST-" "L03-2-CYCLE TEST-" "L03-2-T-RISE TEST-"] -> w1485
                                frame "CHART TEST", Default {
                                }
                                frame "CYCLE TEST" {
                                }
                                frame "T-RISE TEST" {
                                }
                                }
